vi "drivetrain_create.vi"(11 "Robot":T1) -> ()   [LabVIEW 2011]
uses:
  Robot Ctl.ctl
  <vilib>/Rock Robotics/SystemInterfaces/Typedef/FPGA_TypedefDigitalModule.ctl
  <vilib>/Rock Robotics/SystemInterfaces/DIO/FPGA_DIOPWMChannel.ctl
  <vilib>/Rock Robotics/SystemInterfaces/DIO/FPGA_DIOChannel.ctl
  <vilib>/Rock Robotics/SystemInterfaces/Typedef/FPGA_TypedefAnalogModuleForGyro.ctl
  <vilib>/Rock Robotics/WPI/Encoder/WPI_EncoderType.ctl
  <vilib>/Rock Robotics/WPI/SafetyOutput/WPI_SafetyOutputConfigMenu.ctl
  <vilib>/Rock Robotics/SystemInterfaces/AI/FPGA_AIGyroChannel.ctl
  <vilib>/Rock Robotics/WPI/Counter/WPI_CounterDigitalInputToDigitalSource.vi
  <vilib>/Rock Robotics/WPI/RobotDrive/WPI_RobotDriveOpen2MotorWithVictor.vi
panel:
  out "pitch cal":dbl
  out "yaw cal":dbl
  # "Create Drivetrain\n\nThis VI opens all of the refnums that Drivetrain requires"
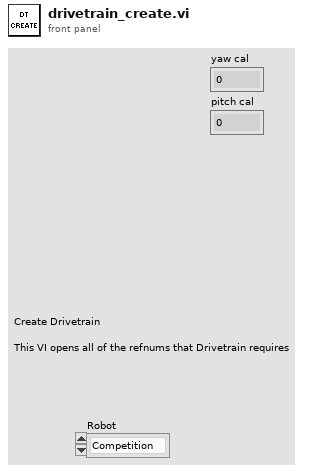
[diagram p1: front panel]
types:
  T1 = typedef "Robot Ctl.ctl" = enum16{"Competition", "Practice"}
  T2 = typedef "WPI_SafetyOutputConfigMenu.ctl" = enum16{"Enable", "Disable"}
  T3 = typedef "WPI_EncoderType.ctl" = enum16{"1x", "2x", "4x"}
  T4 = typedef "FPGA_DIOPWMChannel.ctl" = enum8{"PWM 1", "PWM 2", "PWM 3", "PWM 4", "PWM 5", "PWM 6", "PWM 7", "PWM 8", "PWM 9", "PWM 10", "Invalid"}
  T5 = typedef "FPGA_TypedefAnalogModuleForGyro.ctl" = enum16{"Analog Module 1"}
  T6 = typedef "FPGA_DIOChannel.ctl" = enum8{"DIO 1", "DIO 2", "DIO 3", "DIO 4", "DIO 5", "DIO 6", "DIO 7", "DIO 8", "DIO 9", "DIO 10", "DIO 11", "DIO 12", "DIO 13", "DIO 14", "Invalid"}
  T7 = typedef "FPGA_TypedefDigitalModule.ctl" = enum16{"Digital Module 1", "Digital Module 2"}
  T8 = typedef "FPGA_AIGyroChannel.ctl" = enum8{"AI 1", "AI 2", "Invalid"}
  T9 = typedef "WPI_GyroDevRef.ctl" = cluster{"DevStatus":errorcluster, "Analog Module":T10, "Analog Channel":T11, "Offset":dbl, "Gain (VoltsPerDegree/Second)":dbl}
  T10 = typedef "FPGA_TypedefAnalogModule.ctl" = enum16{"Analog Module 1", "Analog Module 2"}
  T11 = typedef "FPGA_AIChannel.ctl" = enum8{"AI 1", "AI 2", "AI 3", "AI 4", "AI 5", "AI 6", "AI 7", "AI 8", "Invalid"}
  T12 = typedef "WPI_DigitalInputDevRef.ctl" = cluster{"DevStatus":errorcluster, "DIO Channel":T6, "Digital Module":T7}
  T13 = typedef "FPGA_CounterEncoderSourceConvertionLVSourceType.ctl" = cluster{"DevStatus":errorcluster, "AnalogTriggerMode?":bool, "DigitalMode":cluster{"Digital Module":T7, "DIO Channel":T14}, "AnalogTriggerMode":cluster{"AnalogTriggerIndex":T15, "OutputType":T16}}
  T14 = typedef "FPGA_DIODigitalSourceChannel.ctl" = enum8{"DIO 1", "DIO 2", "DIO 3", "DIO 4", "DIO 5", "DIO 6", "DIO 7", "DIO 8", "DIO 9", "DIO 10", "DIO 11", "DIO 12", "DIO 13", "DIO 14", "Disabled"}
  T15 = typedef "FPGA_AnalogTriggerIndex.ctl" = enum8{"Trig 0", "Trig 1", "Trig 2", "Trig 3", "Trig 4", "Trig 5", "Trig 6", "Trig 7", "Invalid"}
  T16 = typedef "FPGA_AnalogTriggerOutType.ctl" = enum16{"InWindow", "TriggerState", "Rising", "Falling"}
  T17 = typedef "WPI_ServoDeviceRef.ctl" = cluster{"DeviceStatus":errorcluster, "Digital Module":T7, "PWM Channel":T4, "DeadBand":T18}
  T18 = typedef "WPI_PWMDeadband.ctl" = cluster{"Name":string, "maxPositivePwm":i32, "minPositivePwm":i32, "centerPwm":i32, "maxNegativePwm":i32, "minNegativePwm":i32, "angularRange":u16}
  T19 = typedef "WPI_EncoderDevRef.ctl" = cluster{"DevStatus":errorcluster, "EncoderIndex":T20, "CounterIndex":T21, "DistancePerCount":dbl, "Decoding Type":T3}
  T20 = typedef "FPGA_EncoderIdx.ctl" = enum8{"Enc 0", "Enc 1", "Enc 2", "Enc 3", "Invalid"}
  T21 = typedef "FPGA_CounterCtrSystemIndex.ctl" = enum8{"Ctr 0", "Ctr 1", "Ctr 2", "Ctr 3", "Ctr 4", "Ctr 5", "Ctr 6", "Ctr 7", "Invalid"}
  T22 = typedef "WPI_RobotDriveDevRef.ctl" = cluster{"DevStatus":errorcluster, "Motors[]":T23[], "Square Inputs":bool, "Max Output":dbl}
  T23 = typedef "WPI_MotorControlDeviceRef.ctl" = cluster{"DeviceStatus":errorcluster, "Type":enum16{"PWM", "CAN"}, "PWM":cluster{"Digital Module":T7, "PWM Channel":T4, "DeadBand":T18}, "CAN":cluster{"Device Number":u8, "Control Mode":T24, "Semaphore":T25, "Max Vout":dbl}, "Invert":bool, "TransformRef":T26, "InvTransformRef":T26}
  T24 = typedef "WPI_CANJaguar_ControlMode.ctl" = enum8{"Percent VBus", "Current", "Speed", "Position", "Voltage"}
  T25 = typedef "Semaphore RefNum" = refnum<k1>
  T26 = typedef "WPI_PWMTransform_ConPane.ctl" = refnum<vi>
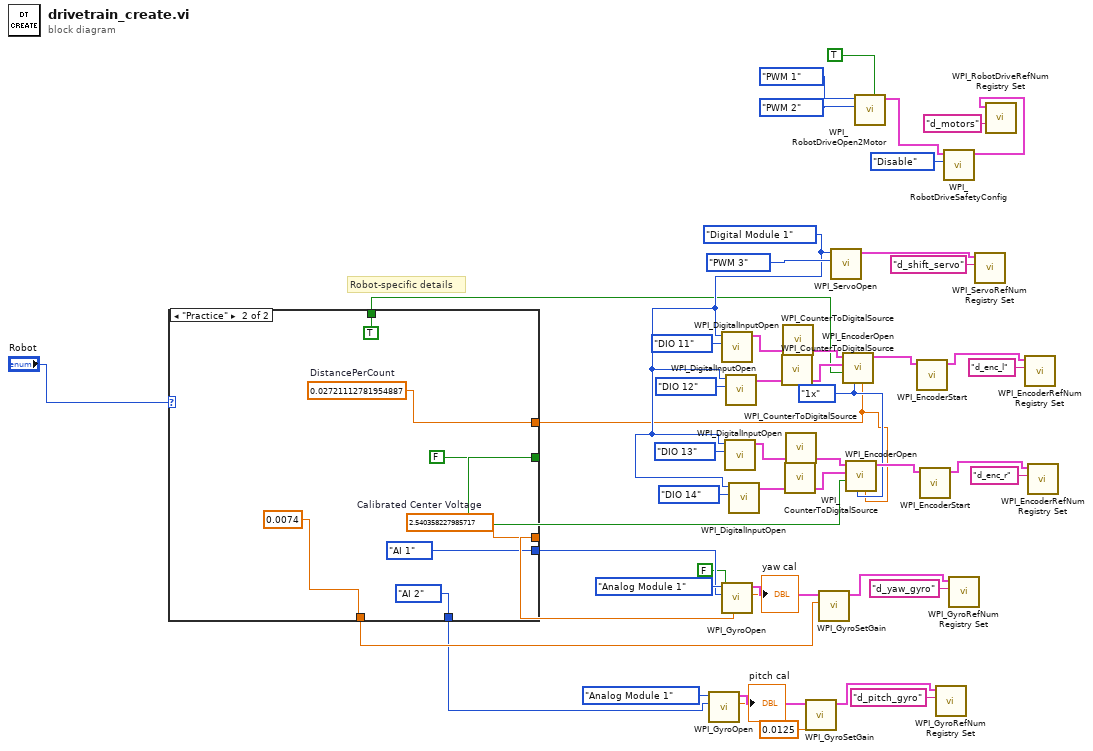
[diagram p0: block diagram]
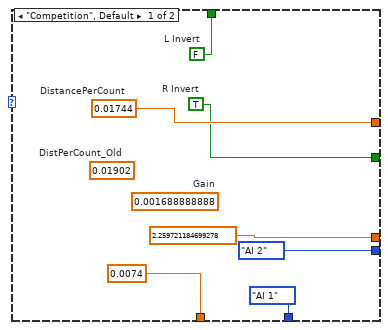
[diagram p2: hidden frame]
diagram:
  w13 = WPI_EncoderType."1x" ("Decoding Type")
  w28 = FPGA_TypedefDigitalModule."Digital Module 1" ("Digital Module (Module 1)")
  # "Robot-specific details"
  n1 = case shown="\"Practice\"" "Robot" {
    tunnel: [w57 TRUE ("L Invert")] -> w11
    tunnel: [w56 w61] -> w10
    tunnel: [w55 FALSE ("R Invert")] -> w9
    tunnel: [0.0074 ("DistancePerCount") 0.0074 ("DistancePerCount")] -> w8
    tunnel: [FPGA_AIGyroChannel."AI 1" ("Analog Channel") FPGA_AIGyroChannel."AI 2" ("Analog Channel")] -> w4
    tunnel: [FPGA_AIGyroChannel."AI 2" ("Analog Channel") FPGA_AIGyroChannel."AI 1" ("Analog Channel")] -> w3
    tunnel: [2.259721184699278 ("Calibrated Center Voltage") w58] -> w1
    frame "Competition", Default {
      (unwired) 0.01902  # DistPerCount_Old
      (unwired) 0.001688888888  # Gain
      w55 = TRUE  # R Invert
      w57 = FALSE  # L Invert
      w56 = 0.01744  # DistancePerCount
    }
    frame "Practice" {
      w58 = 2.540358227985717  # Calibrated Center Voltage
      w61 = 0.02721112781954887  # DistancePerCount
    }
  }
  n2 = call <vilib>:"WPI_GyroOpen.vi"("Analog Channel"=w4, "Analog Module (Module 1)"=FPGA_TypedefAnalogModuleForGyro."Analog Module 1") -> ("Calibrated Center Voltage Out"=→"pitch cal":dbl, "GyroDevRef"=w21:T9)  [unwired: 7 in, 1 out]
  n3 = call <vilib>:"WPI_DigitalInputOpen.vi"("DIO Channel"=FPGA_DIOChannel."DIO 11", "Digital Module (Module 1)"=w28) -> ("DigitalInputDevRef"=w40:T12)  [unwired: 8 in, 1 out]
  n4 = call <vilib>:"WPI_GyroOpen.vi"("Calibrated Center Voltage"=w1, "Calibrate On Open"=FALSE, "Analog Channel"=w3, "Analog Module (Module 1)"=FPGA_TypedefAnalogModuleForGyro."Analog Module 1") -> ("Calibrated Center Voltage Out"=→"yaw cal":dbl, "GyroDevRef"=w25:T9)  [unwired: 5 in, 1 out]
  n5 = call <vilib>:"WPI_DigitalInputOpen.vi"("DIO Channel"=FPGA_DIOChannel."DIO 13", "Digital Module (Module 1)"=w28) -> ("DigitalInputDevRef"=w31:T12)  [unwired: 8 in, 1 out]
  n6 = call <vilib>:"WPI_DigitalInputOpen.vi"("DIO Channel"=FPGA_DIOChannel."DIO 12", "Digital Module (Module 1)"=w28) -> ("DigitalInputDevRef"=w38:T12)  [unwired: 8 in, 1 out]
  n7 = call <vilib>:"WPI_DigitalInputOpen.vi"("DIO Channel"=FPGA_DIOChannel."DIO 14", "Digital Module (Module 1)"=w28) -> ("DigitalInputDevRef"=w29:T12)  [unwired: 8 in, 1 out]
  n8 = call-poly <vilib>:"WPI_CounterToDigitalSource.vi"("DigitalInputDevRef"=w38) -> ("Digital Source"=w45:T13)  [unwired: 6 in]
  n9 = call-poly <vilib>:"WPI_CounterToDigitalSource.vi"("DigitalInputDevRef"=w40) -> ("Digital Source"=w44:T13)  [unwired: 6 in]
  n10 = call-poly <vilib>:"WPI_CounterToDigitalSource.vi"("DigitalInputDevRef"=w29) -> ("Digital Source"=w36:T13)  [unwired: 6 in]
  n11 = call-poly <vilib>:"WPI_CounterToDigitalSource.vi"("DigitalInputDevRef"=w31) -> ("Digital Source"=w35:T13)  [unwired: 6 in]
  n12 = call <vilib>:"WPI_GyroSetGain.vi"("Gain (VoltsPerDegree/Second)"=0.0125, "GyroDevRef"=w21) -> ("GyroDevRef"=w20:T9)  [unwired: 8 in, 1 out]
  n13 = call <vilib>:"WPI_GyroSetGain.vi"("Gain (VoltsPerDegree/Second)"=w8, "GyroDevRef"=w25) -> ("GyroDevRef"=w24:T9)  [unwired: 8 in, 1 out]
  n14 = call <vilib>:"WPI_ServoOpen.vi"("PWM Channel"=FPGA_DIOPWMChannel."PWM 3", "Digital Module (Module 1)"=w28) -> ("ServoDeviceRef"=w48:T17)  [unwired: 8 in, 1 out]
  n15 = call <vilib>:"WPI_EncoderOpen.vi"("DistancePerCount"=w10, "Decoding Type"=w13, "Invert Direction (False)"=w11, "BSource"=w45, "ASource"=w44) -> ("EncoderDevRef"=w43:T19)  [unwired: 5 in, 1 out]
  n16 = call <vilib>:"WPI_EncoderOpen.vi"("DistancePerCount"=w10, "Decoding Type"=w13, "Invert Direction (False)"=w9, "BSource"=w36, "ASource"=w35) -> ("EncoderDevRef"=w34:T19)  [unwired: 5 in, 1 out]
  n17 = call-poly <vilib>:"WPI_RobotDriveOpen2Motor.vi"("Right Motor Inverted"=TRUE, "Right Motor"=FPGA_DIOPWMChannel."PWM 2", "Left Motor"=FPGA_DIOPWMChannel."PWM 1") -> ("RobotDriveDevRef"=w7:T22)  [unwired: 7 in, 1 out]
  n18 = call <vilib>:"WPI_EncoderStart.vi"("EncoderDevRef"=w43) -> ("EncoderDevRef"=w42:T19)  [unwired: 9 in, 1 out]
  n19 = call <vilib>:"WPI_EncoderStart.vi"("EncoderDevRef"=w34) -> ("EncoderDevRef"=w33:T19)  [unwired: 9 in, 1 out]
  n20 = call <vilib>:"WPI_GyroRefNum Registry Set.vi"("refnum name"="d_pitch_gyro", "GyroDevRef"=w20) -> ()  [unwired: 8 in, 2 out]
  n21 = call <vilib>:"WPI_RobotDriveSafetyConfig.vi"("mode"=WPI_SafetyOutputConfigMenu."Disable", "RobotDriveDevRef"=w7) -> ("RobotDriveDevRef"=w6:T22)  [unwired: 8 in, 1 out]
  n22 = call <vilib>:"WPI_GyroRefNum Registry Set.vi"("refnum name"="d_yaw_gyro", "GyroDevRef"=w24) -> ()  [unwired: 8 in, 2 out]
  n23 = call <vilib>:"WPI_ServoRefNum Registry Set.vi"("refnum name"="d_shift_servo", "ServoDeviceRef"=w48) -> ()  [unwired: 8 in, 2 out]
  n24 = call <vilib>:"WPI_RobotDriveRefNum Registry Set.vi"("refnum name"="d_motors", "RobotDriveDevRef"=w6) -> ()  [unwired: 8 in, 2 out]
  n25 = call <vilib>:"WPI_EncoderRefNum Registry Set.vi"("refnum name"="d_enc_l", "EncoderDevRef"=w42) -> ()  [unwired: 8 in, 2 out]
  n26 = call <vilib>:"WPI_EncoderRefNum Registry Set.vi"("refnum name"="d_enc_r", "EncoderDevRef"=w33) -> ()  [unwired: 8 in, 2 out]
